vi "test O grid.vi"() -> ()   [LabVIEW 2010]
panel:
  in  "stop":bool
  out "XY":cluster{"Direction":dbl[], "Magnitude":dbl[]}(graph)
  out "After":dbl[][](graph)
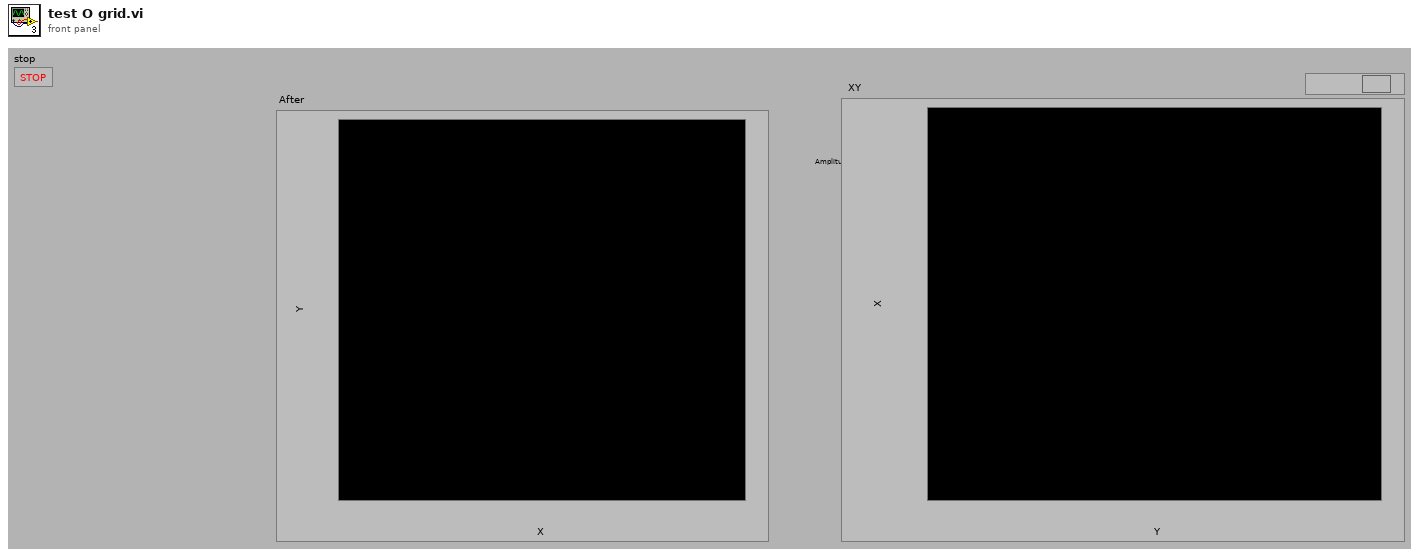
[diagram p1: front panel]
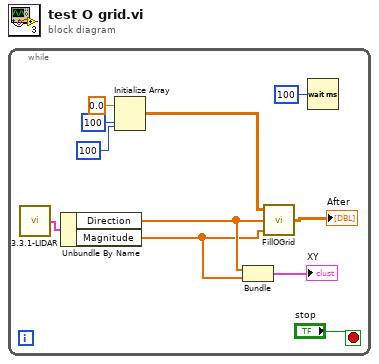
[diagram p0: block diagram]
diagram:
  n1 = while {
    stop <- "stop" stop-if-true
    n2 = call "3.3.1-LIDAR.vi"() -> ("XY"=w4:cluster{"Direction":dbl[], "Magnitude":dbl[]})
    n3 = Unbundle By Name(w4) -> ("Direction"=w3:dbl[], "Magnitude"=w2:dbl[])
    n4 = Initialize Array(0.0 ("element"), 100 ("dimension size"), 100 ("dimension size")) -> (w8:dbl[][])
    n5 = Bundle("Direction"=w3, "Magnitude"=w2) -> (→"XY":cluster{"Direction":dbl[], "Magnitude":dbl[]})  [unwired: 1 in]
    n6 = call "FillOGrid.vi"("Y"=w2, "X"=w3, "OGrid In"=w8) -> ("OGrid Out"=→"After":dbl[][])
    n7 = Wait (ms)(milliseconds to wait=u32 100) -> ()  [unwired: 1 out]
  }
